vi "Create Enum Accessor.vi"(8 "error in (no error)":errorcluster, 10 "Message Name":string, 11 "Library":refnum<vi>) -> (0 "error out":errorcluster, 3 "Library":refnum<vi>)   [LabVIEW 2019, in "gRPC Template Creation Utility.lvlib"]
uses:
  gRPC Template Creation Utility.lvlib
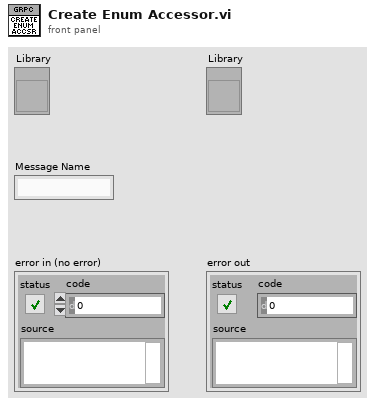
[diagram p1: front panel]
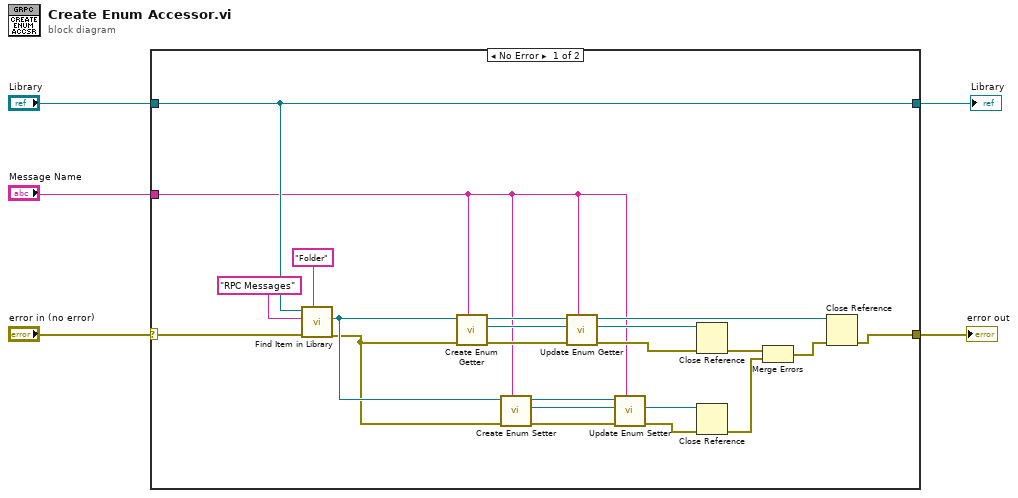
[diagram p0: block diagram]
diagram:
  n1 = case shown="No Error" "error in (no error)" {
    selector: "error in (no error)" -> [w21 w28]
    tunnel: "Library" -> [w20 w29]
    tunnel: "Message Name" -> [w8 _]
    tunnel: [w22 w28] -> w4
    tunnel: [w20 w29] -> w2
    frame No Error {
      n2 = call "Find Item in Library.vi"("Item Type"="Folder", "error in (no error)"=w21, "Item Name"="RPC Messages", "Library item in"=w20) -> ("error out"=w18:errorcluster, "Project Item (Library Item)"=w19:refnum<vi>)  [unwired: 4 in, 2 out]
      n3 = call "Create Enum Getter.vi"("RPC Message Name"=w8, "error in (no error)"=w18, "RPC Messages Folder (ProjectItem) in"=w19) -> ("error out"=w15:errorcluster, "Message Getter out"=w16:refnum<vi>, "RPC Messages Folder (ProjectItem) out"=w17:refnum<vi>)  [unwired: 6 in]
      n4 = call "Create Enum Setter.vi"("RPC Message Name"=w8, "error in (no error)"=w18, "RPC Messages Folder (ProjectItem) in"=w19) -> ("error out"=w9:errorcluster, "Message Setter out"=w10:refnum<vi>, "RPC Messages Folder (ProjectItem) out"=w11:refnum<vi>)  [unwired: 6 in]
      n5 = call "Update Enum Getter.vi"("RPC Message Name"=w8, "error in (no error)"=w15, "Message Getter in"=w16, "RPC Messages Folder (ProjectItem) in"=w17) -> ("error out"=w14:errorcluster, "Message Getter out"=w13:refnum<vi>, "RPC Messages Folder (ProjectItem) out"=w12:refnum<vi>)  [unwired: 5 in]
      n6 = call "Update Enum Setter.vi"("RPC Message Name"=w8, "error in (no error)"=w9, "Message Getter in"=w10, "RPC Messages Folder (ProjectItem) in"=w11) -> ("error out"=w7:errorcluster, "Message Getter out"=w6:refnum<vi>)  [unwired: 5 in, 1 out]
      n7 = Close Reference(reference=w13, error in (no error)=w14) -> (error out=w25:errorcluster)
      n8 = Close Reference(reference=w6, error in (no error)=w7) -> (error out=w24:errorcluster)
      n9 = Merge Errors(w25, w24) -> (w23:errorcluster)
      n10 = Close Reference(reference=w12, error in (no error)=w23) -> (error out=w22:errorcluster)
    }
    frame Error {
    }
  }
  "error out" <- w4
  "Library" <- w2
